vi "3.3.1-LIDAR.vi"() -> (0 "XY":cluster{"Direction":dbl[], "Magnitude":dbl[]}(graph))   [LabVIEW 2010]
uses:
  4-High Neurons/4.0-Timing Badass.ctl
  _typedefs/3.3.1-LIDAR Data Typedef.ctl
  <instrlib>/Hokuyo URG Series/Public/Initialize-Standard.vi
  3.0-Global.vi
  <instrlib>/Hokuyo URG Series/Hokuyo URG Series.lvlib
panel:
  out "HB":T1
  out "Queue overflow?":bool
  out "XY Rotated":cluster{"Direction":dbl[], "Magnitude":dbl[]}(graph)
  out "size(s)":i32
  out "\"Polar\"":cluster{"Direction":dbl[], "Magnitude":dbl[]}(graph)
  out "Angle Array":dbl[](array[numeric])
  out "Magnitude Array":dbl[](array[numeric])
  in  "ID Query?":bool
  in  "Stop":bool
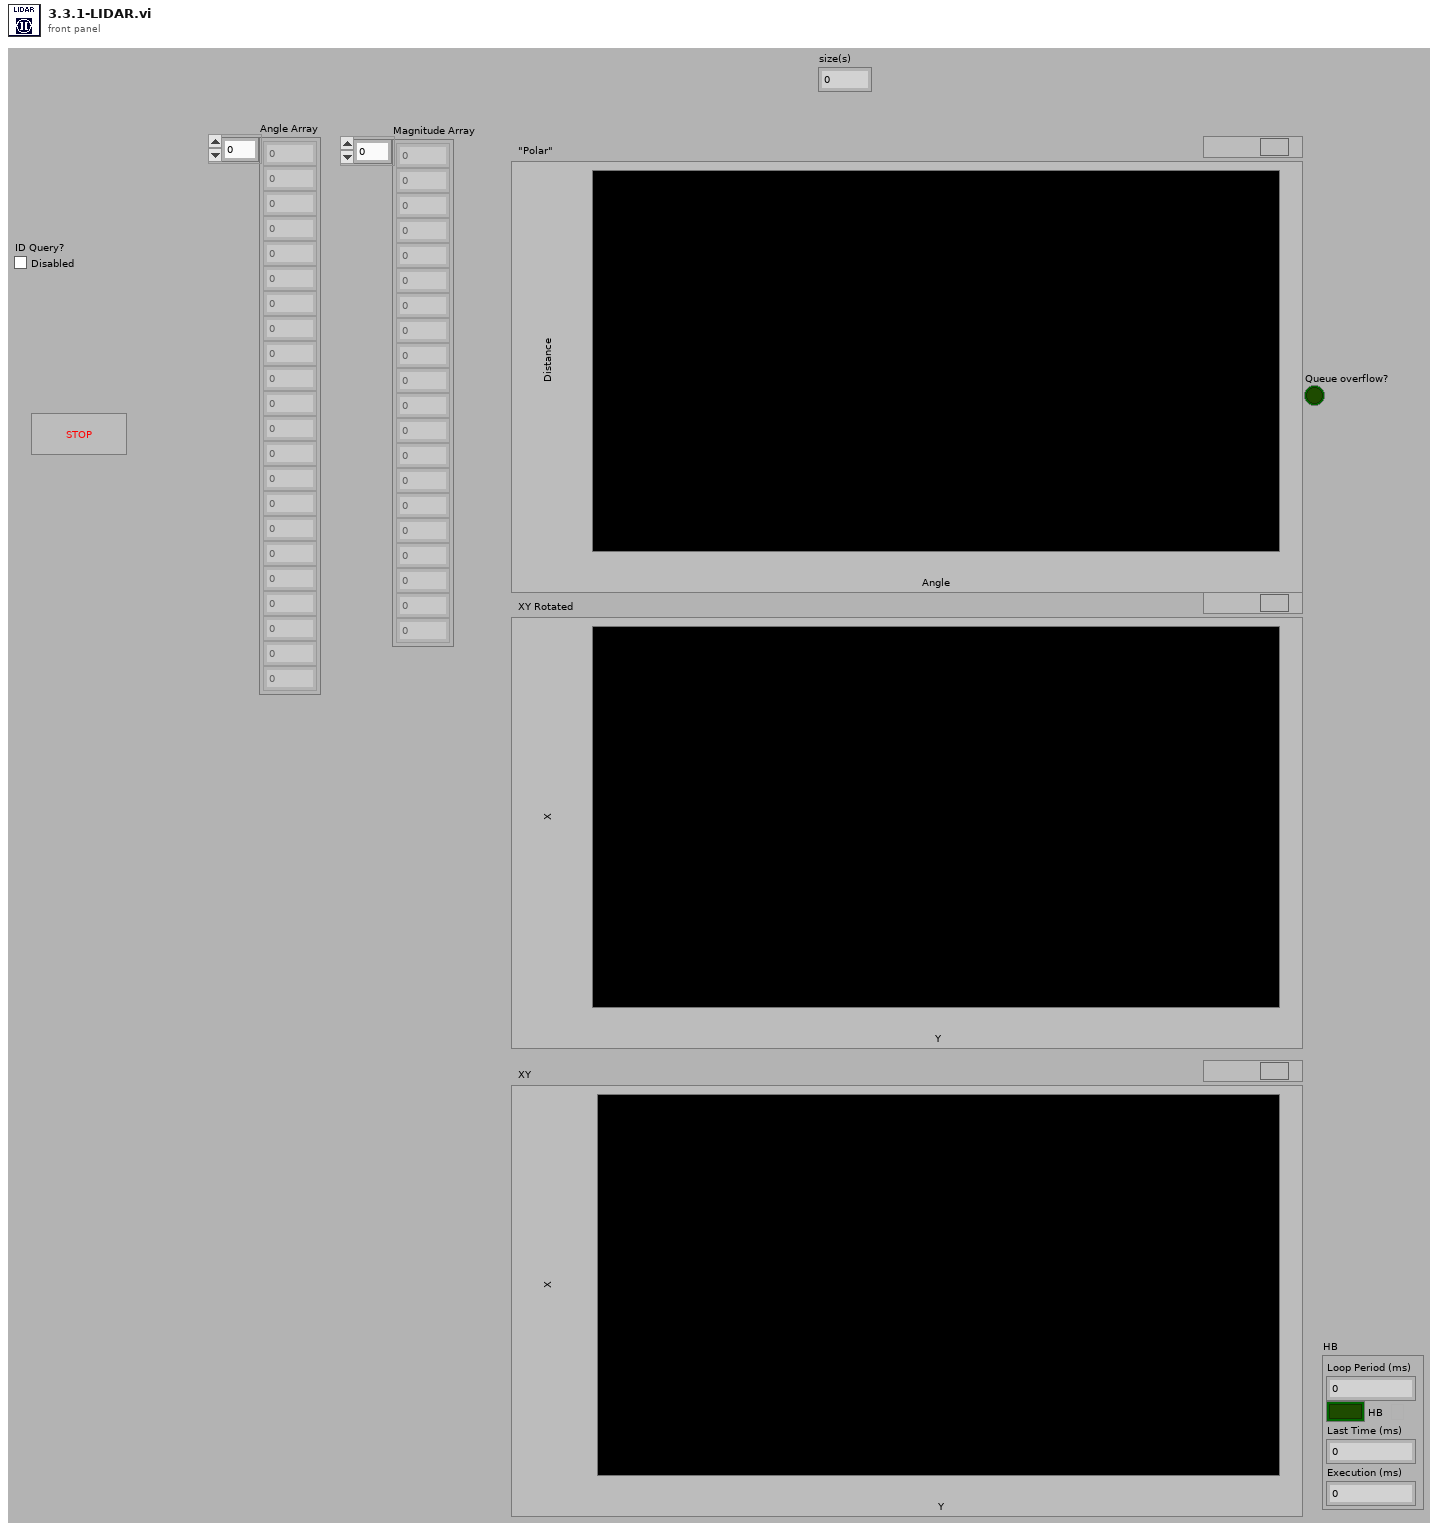
[diagram p1: front panel]
types:
  T1 = typedef "4.0-Timing Badass.ctl" = cluster{"Loop Period (ms)":u32, "HB":bool, "Last Time (ms)":u32, "Execution (ms)":u32}
  T2 = typedef "3.3.1-LIDAR Data Typedef.ctl" = cluster{"Angle array":dbl[], "Magnitude array ":dbl[]}
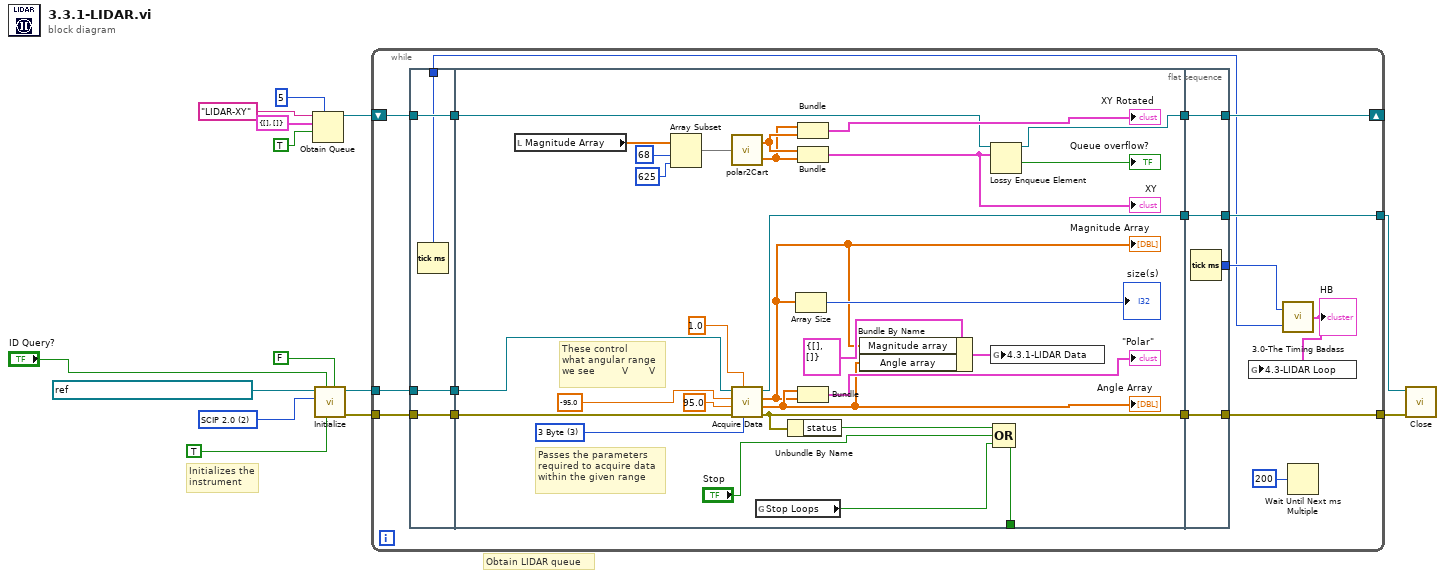
[diagram p0: block diagram]
diagram:
  w7 = u32 2 items=["Convert to Latest", "SCIP 1.1", "SCIP 2.0", "SCIP 2.2"] ("Protocol (2: SCIP 2.0)")
  # "Obtain LIDAR queue"
  # "Initializes the instrument"
  n1 = Obtain Queue(max queue size (-1, unlimited)=5, name (unnamed)="LIDAR-XY", element data type=cluster{"X":dbl[], "Y":dbl[]} {"X"=[], "Y"=[]} ("output cluster"), create if not found? (T)=TRUE) -> (queue out=w6:refnum<queue>)  [unwired: 1 in, 2 out]
  n2 = call-poly <instrlib>:"Initialize.vi"("Reset? (F: No)"=FALSE ("Reset Instrument (Disabled)"), "Checksum (Disabled)"=TRUE ("Checksum"), "ID Query? (Enabled)"="ID Query?", "Protocol (2: SCIP 2.0)"=w7, "VISA resource name"=refnum<visa-resource-name> "TCPIP::10.10.10.15::10940::Socket") -> ("error out"=w8:errorcluster, "VISA resource name out"=w9:refnum<visa-resource-name>)  [unwired: 5 in]
  n3 = while {
    tunnel: w9 -> [w30]
    tunnel: [w27] -> w14
    tunnel: [w28] -> w10
    tunnel: w8 -> [w29]
    shift-right: [w26] -> _
    shift-left: w6 -> [w25]
    stop <- w31 stop-if-true
    n4 = flat-sequence {
      tunnel: w25 -> [w33]
      tunnel: w29 -> [w34]
      tunnel: w30 -> [w35]
      tunnel: [w35] -> w24
      tunnel: [w34] -> w23
      tunnel: [w33] -> w22
      tunnel: [w32] -> w17
      tunnel: [w62] -> w31
      tunnel: w24 -> [w58]
      tunnel: w23 -> [w57]
      tunnel: w22 -> [w42]
      tunnel: [w55] -> w21
      tunnel: [w54] -> w20
      tunnel: [w43] -> w19
      tunnel: [w66] -> w26
      tunnel: [w67] -> w27
      tunnel: [w68] -> w28
      tunnel: w21 -> [w68]
      tunnel: w20 -> [w67]
      tunnel: w19 -> [w66]
      tunnel: [w65] -> w18
      frame #0 {
        n5 = Tick Count (ms)() -> (millisecond timer value=w32:u32)
      }
      frame #1 {
        w56 = u16 3 items=["2 Byte"=2, "3 Byte"=3] ("Encoding Width")
        # "These control\nwhat angular range\nwe see         V       V"
        # "Passes the parameters\nrequired to acquire data\nwithin the given range"
        n6 = local read "Magnitude Array"() -> (w37:dbl[])
        n7 = Array Subset(array=w37, index=68 ("length"), length=625) -> (w36:dbl[])
        n8 = call "polar2Cart.vi"("Magnitudes"=w36) -> ("X"=w45:dbl[], "Y"=w44:dbl[])
        n9 = call <instrlib>:"Acquire Data.vi"("Data Encoding Width (3 Byte)"=w56, "Cluster Count (1)"=1.0 ("Cluster Count"), "error in (no error)"=w57, "End Point (120°)"=95.0 ("End Point"), "Start Point (-120°)"=-95.0 ("Start Point"), "VISA resource name"=w58) -> ("error out"=w54:errorcluster, "Direction"=w49:dbl[], "Magnitude"=w47:dbl[], "VISA resource name out"=w55:refnum<visa-resource-name>)  [unwired: 2 in]
        "Magnitude Array" <- w47
        "Angle Array" <- w49
        n10 = global read "3.0-Global.vi" "Stop Loops"() -> (w51:bool)
        n11 = Unbundle By Name(w54) -> ("status"=w64:bool)
        n12 = Array Size(array=w47) -> (size(s)=→"size(s)":i32)
        n13 = Bundle("Y"=w44, "X"=w45) -> (→"XY Rotated":cluster{"Y":dbl[], "X":dbl[]})  [unwired: 1 in]
        n14 = Bundle("X"=w45, "Y"=w44) -> (w40:cluster{"X":dbl[], "Y":dbl[]})  [unwired: 1 in]
        "XY" <- w40
        n15 = Bundle("Direction"=w49, "Magnitude"=w47) -> (→"\"Polar\"":cluster{"Direction":dbl[], "Magnitude":dbl[]})  [unwired: 1 in]
        n16 = Bundle By Name(cluster=T2 {"Angle array"=[], "Magnitude array "=[]} ("LIDAR Data"), "Magnitude array"=w47, "Angle array"=w49) -> (w52:T2)
        n17 = Lossy Enqueue Element(queue=w42, element=w40) -> (queue out=w43:refnum<queue>, overflow?=→"Queue overflow?":bool)  [unwired: 1 in, 2 out]
        n18 = global write "3.0-Global.vi" "4.3.1-LIDAR Data"(w52) -> ()
        n19 = Compound Arithmetic op=OR(w64, "Stop", w51) -> (w62:bool)
      }
      frame #2 {
        n20 = Tick Count (ms)() -> (millisecond timer value=w65:u32)
      }
    }
    n21 = call "3.0-The Timing Badass.vi"("Start"=w17, "End"=w18) -> ("Super Heart Beat"=w15:T1)
    "HB" <- w15
    n22 = global write "3.0-Global.vi" "4.3-LIDAR Loop"(w15) -> ()
    n23 = Wait Until Next ms Multiple(millisecond multiple=u32 200) -> ()  [unwired: 1 out]
  }
  n24 = call <instrlib>:"Close.vi"("error in (no error)"=w14, "VISA resource name"=w10) -> ()  [unwired: 9 in, 1 out]
